vi "Initialize.vi"(2 "error in":errorcluster, 3 "VISA arduino in":refnum<visa-resource-name>) -> (0 "error out":errorcluster, 1 "VISA arduino out":refnum<visa-resource-name>)   [LabVIEW 2021]
uses:
  Delay_Global.vi
  <vilib>/Instr/_visa.llb/VISA Configure Serial Port (Instr).vi
  <vilib>/Utility/error.llb/Error Cluster From Error Code.vi
  <vilib>/ErrorRing/Error Ring.xnode
panel:
  out "delay":u32
  out "read buffer":string
  out "ext delay":u32
  out "max iterator":u8
  # "Private"
  # "Public"
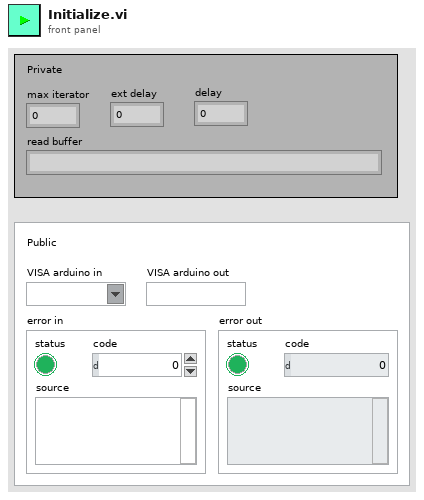
[diagram p1: front panel]
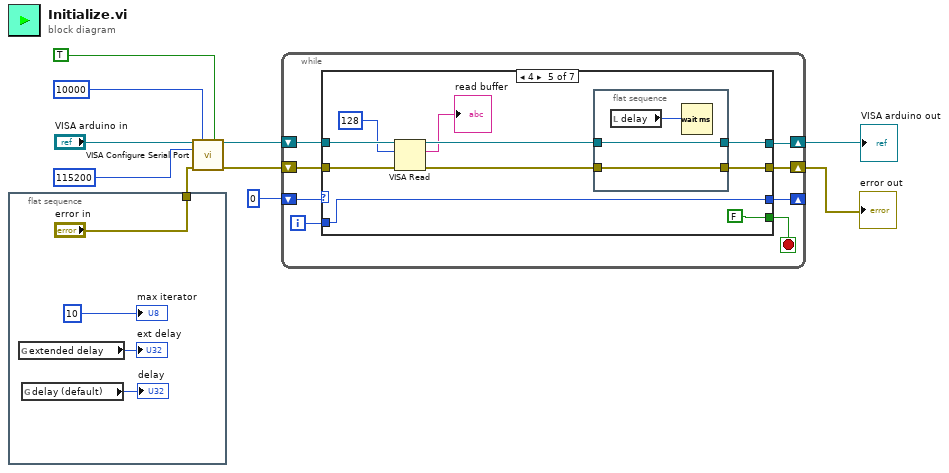
[diagram p0: block diagram]
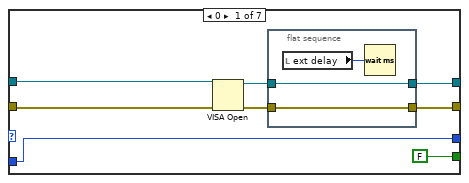
[diagram p2: hidden frame]
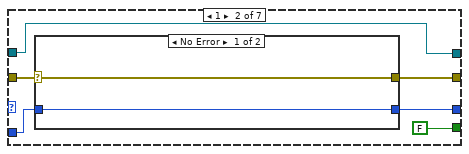
[diagram p3: hidden frame]
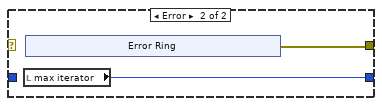
[diagram p4: hidden frame]
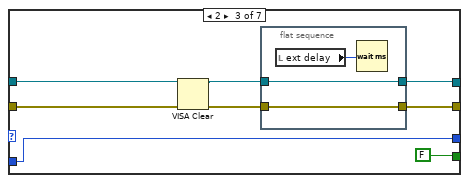
[diagram p5: hidden frame]
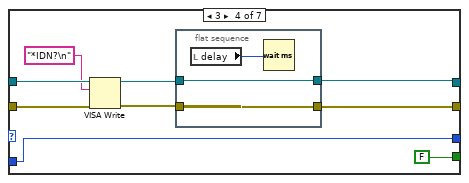
[diagram p6: hidden frame]
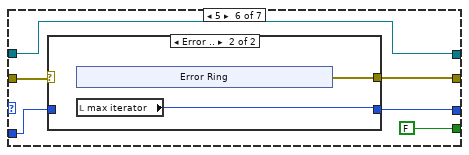
[diagram p7: hidden frame]
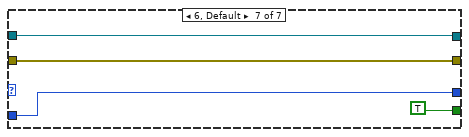
[diagram p9: hidden frame]
diagram:
  n1 = flat-sequence {
    tunnel: ["error in"] -> w3
    frame #0 {
      n2 = global read "Delay_Global.vi" "extended delay"() -> (→"ext delay":u32)
      n3 = global read "Delay_Global.vi" "delay (default)"() -> (→"delay":u32)
      "max iterator" <- u8 10 ("Numeric")
    }
  }
  n4 = call-poly "VISA Configure Serial Port"("VISA resource name"="VISA arduino in", "timeout (10sec)"=u32 10000, "Enable Termination\nChar (T)"=TRUE ("Enable Termination\nChar (T)"), "baud rate (9600)"=u32 115200, "error in (no error)"=w3) -> ("VISA resource name out"=w7:refnum<visa-resource-name>, "error out"=w6:errorcluster)  [unwired: 9 in]
  n5 = while {
    shift-right: [w20] -> w1
    shift-left: w7 -> [w22]
    shift-right: [w19] -> w2
    shift-left: w6 -> [w21]
    shift-right: [w16] -> _
    shift-left: 0 -> [w18]
    i -> [w17]
    stop <- w15 stop-if-true
    n6 = case shown="4" w18 {
      tunnel: w22 -> [w30 w37 w56 w68 w81 w87 w103]
      tunnel: w21 -> [w29 w39 w55 w67 w80 w89 w102]
      tunnel: [w26 w37 w52 w61 w76 w87 w103] -> w20
      tunnel: [w24 w38 w50 w63 w74 w88 w102] -> w19
      tunnel: w17 -> [w28 w35 w54 w65 w78 w85 w101]
      tunnel: [w28 w36 w54 w65 w78 w86 w101] -> w16
      tunnel: [FALSE ("Enable Termination\nChar (T)") FALSE ("Enable Termination\nChar (T)") FALSE ("Enable Termination\nChar (T)") FALSE ("Enable Termination\nChar (T)") FALSE ("Enable Termination\nChar (T)") FALSE ("Enable Termination\nChar (T)") TRUE ("Enable Termination\nChar (T)")] -> w15
      frame 0 {
        n7 = VISA Open(error in (no error)=w29, VISA resource name=w30) -> (VISA resource name=w25:refnum<visa-resource-name>, error out=w23:errorcluster)  [unwired: 3 in]
        n8 = flat-sequence {
          tunnel: [w33] -> w26
          tunnel: w25 -> [w33]
          tunnel: [w32] -> w24
          tunnel: w23 -> [w32]
          frame #0 {
            n9 = local read "ext delay"() -> (w31:u32)
            n10 = Wait (ms)(milliseconds to wait=w31) -> ()  [unwired: 1 out]
          }
        }
      }
      frame 1 {
        n11 = case shown="No Error" w39 {
          selector: w39 -> [w41 _]
          tunnel: [w41 w42] -> w38
          tunnel: [w40 w43] -> w36
          tunnel: w35 -> [w40 _]
          frame No Error {
          }
          frame Error {
            n12 = local read "max iterator"() -> (w43:u8)
            n13 = xnode "Error Ring"() -> ("error out"=w42:errorcluster)
          }
        }
      }
      frame 2 {
        n14 = VISA Clear(VISA resource name=w56, error in (no error)=w55) -> (VISA resource name out=w51:refnum<visa-resource-name>, error out=w49:errorcluster)
        n15 = flat-sequence {
          tunnel: [w59] -> w52
          tunnel: w51 -> [w59]
          tunnel: [w58] -> w50
          tunnel: w49 -> [w58]
          frame #0 {
            n16 = local read "ext delay"() -> (w57:u32)
            n17 = Wait (ms)(milliseconds to wait=w57) -> ()  [unwired: 1 out]
          }
        }
      }
      frame 3 {
        n18 = VISA Write(VISA resource name=w68, write buffer="*IDN?\n", error in (no error)=w67) -> (VISA resource name out=w60:refnum<visa-resource-name>, error out=w62:errorcluster)  [unwired: 1 out]
        n19 = flat-sequence {
          tunnel: [w71] -> w63
          tunnel: [w70] -> w61
          tunnel: w62 -> [w71]
          tunnel: w60 -> [w70]
          frame #0 {
            n20 = local read "delay"() -> (w69:u32)
            n21 = Wait (ms)(milliseconds to wait=w69) -> ()  [unwired: 1 out]
          }
        }
      }
      frame 4 {
        n22 = VISA Read(VISA resource name=w81, byte count=u32 128, error in (no error)=w80) -> (VISA resource name out=w75:refnum<visa-resource-name>, read buffer=→"read buffer":string, error out=w73:errorcluster)  [unwired: 1 out]
        n23 = flat-sequence {
          tunnel: [w83] -> w76
          tunnel: w75 -> [w83]
          tunnel: [w82] -> w74
          tunnel: w73 -> [w82]
          frame #0 {
            n24 = local read "delay"() -> (w84:u32)
            n25 = Wait (ms)(milliseconds to wait=w84) -> ()  [unwired: 1 out]
          }
        }
      }
      frame 5 {
        n26 = case shown="Error .." w89 {
          selector: w89 -> [w92 _]
          tunnel: [w92 w94] -> w88
          tunnel: [w91 w93] -> w86
          tunnel: w85 -> [w91 _]
          frame No Error {
          }
          frame Error {
            n27 = xnode "Error Ring"() -> ("error out"=w94:errorcluster)
            n28 = local read "max iterator"() -> (w93:u8)
          }
        }
      }
      frame 6, Default {
      }
    }
  }
  "VISA arduino out" <- w1
  "error out" <- w2
